vi "Send Initialize Force Task.vi"(2 "Task Info In":T1={"Number of Trials"=1, "Sampling Rate (Hz)"=200, "Trial Duration (s)"=10, "Adjusted MVC (N)"=5.0, "R Phase"=0, "L Phase"=0, "L Pattern"=1, "R Pattern"=1, "Time Between Trials (s)"=5, "Lissajous Speed"=200} {"Lissajous Speed" min=1 max=200; "Time Between Trials (s)" min=1 step=1; "R Pattern" min=1 max=20 step=1; "L Pattern" min=1 max=20 step=1; "L Phase" max=360 step=1; "R Phase" max=360 step=1; "Adjusted MVC (N)" min=1.0 step=1.0; "Trial Duration (s)" min=1 step=1; "Sampling Rate (Hz)" min=1 step=1; "Number of Trials" min=1 step=1}, 4 "Scanning?":bool=TRUE, 5 "EMG info":cluster{"Collect EMG?":bool, "EMG Rate":u16}, 6 "DAQ  Channels In":T2={"Force Transducer: Left"="Dev1/ai6", "Force Transducer: Right "="Dev1/ai8", "EMG: Left"="", "EMG: Right"="", "Potentiometer: Left"="", "Potentiometer: Right"=""}, 7 "Priority":T3=enum."Normal" caption="Message Priority (Normal)", 8 "error in (no error)":errorcluster, 9 "TDMS File":refnum<k34>, 10 "Force Calibration Cluster":cluster{"Left":dbl, "Right":dbl}, 11 "Message Enqueuer in":refnum<class "Message Enqueuer.lvclass">) -> (0 "error out":errorcluster, 3 "Message Enqueuer out":refnum<class "Message Enqueuer.lvclass">)   [LabVIEW 2020, in "NI Force Task.lvlib" / "Initialize Force Task Msg.lvclass"]
doc: "Sends the <b>NI Force Task.lvlib:Initialize Force Task Msg.lvclass</b> message.\n\nThis message will call <b>Initialize Force Task.vi</b> on the <b>NI Force Task.lvlib:NI Force Task.lvclass</b> actor.\n\n<b>Initialize Force Task.vi Description</b>"
uses:
  Initialize Force Task Msg.lvclass
  <vilib>/ActorFramework/Message Enqueuer/Message Enqueuer.lvclass
  <vilib>/ActorFramework/Message Enqueuer/Message Priority.ctl
  Task info df.ctl
  C:/Program Files/National Instruments/LabVIEW 2020/vi.lib/ActorFramework/Message/Message.lvclass
  Initialize Force Task Msg.lvclass/Initialize Force Task Msg.ctl
  <vilib>/ActorFramework/Message Enqueuer/Message Enqueuer.lvclass/Message Enqueuer.ctl
  <vilib>/ActorFramework/Message Priority Queue/Priority Enqueue.vi
panel:
  # "Left Arm"
  # "Right Arm"
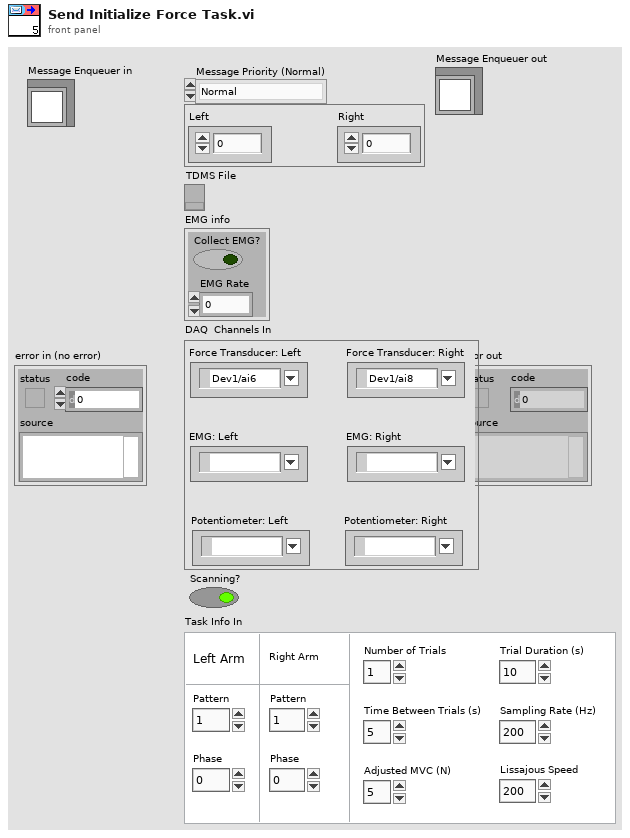
[diagram p1: front panel]
types:
  T1 = typedef "Task info df.ctl" = cluster{"Number of Trials":u8, "Sampling Rate (Hz)":u16, "Trial Duration (s)":u8, "Adjusted MVC (N)":dbl, "R Phase":i32, "L Phase":i32, "L Pattern":u8, "R Pattern":u8, "Time Between Trials (s)":u8, "Lissajous Speed":u16}
  T2 = cluster{"Force Transducer: Left":tag, "Force Transducer: Right ":tag, "EMG: Left":tag, "EMG: Right":tag, "Potentiometer: Left":tag, "Potentiometer: Right":tag}
  T3 = typedef "Actor Framework.lvlib/Message Enqueuer.lvclass/Message Priority.ctl" = enum16{"Low", "Normal", "High"}
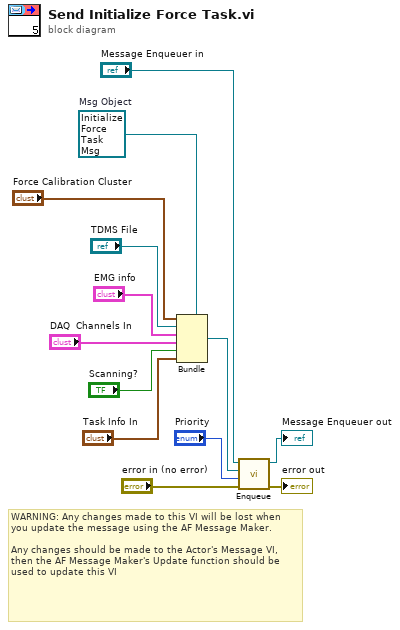
[diagram p0: block diagram]
diagram:
  w7 = refnum<class "Initialize Force Task Msg.lvclass"> refnum  # Msg Object
  # "WARNING: Any changes made to this VI will be lost when you update the message using the AF Message Maker.\n\nAny changes should be made to the Actor's Message VI, then the AF Message Maker's Update function should be used to update this VI"
  n1 = Bundle(cluster=w7, "Force Calibration Cluster", "TDMS File", "EMG info", "DAQ  Channels In", "Scanning?", "Task Info In") -> (w2:refnum<class "Initialize Force Task Msg.lvclass">)
  n2 = call <vilib>:"Enqueue.vi"("error in (no error)"="error in (no error)", "Message Priority (Normal)"="Priority", "Message"=w2, "Message Enqueuer in"="Message Enqueuer in") -> ("error out"=→"error out":errorcluster, "Message Enqueuer out"=→"Message Enqueuer out":refnum<class "Message Enqueuer.lvclass">)  [unwired: 6 in]
